vi "Get Panther Dash Library.vi"() -> (3 "Library out":refnum<vi>)   [LabVIEW 2020, in "Panter Dashboard.lvlib"]
uses:
  Panter Dashboard.lvlib
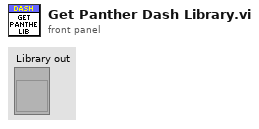
[diagram p1: front panel]
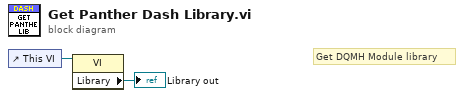
[diagram p0: block diagram]
diagram:
  # "Get DQMH Module library"
  n1 = control-ref of="This VI"() -> (w1:refnum<vi>)
  n2 = property class="VI"(reference=w1) -> ("Library"=→"Library out":refnum<vi>)  [unwired: 1 in, 2 out]
